vi "Get Configured Form Object.vi"(8 "error in (no error)":errorcluster, 10 "Table Name":string, 11 "Form from Table Configuration in":refnum<class "Form from Table Configuration.lvclass">) -> (0 "error out":errorcluster, 2 "Configured Form":refnum<class "Basic Form.lvclass">, 3 "Form from Table Configuration out":refnum<class "Form from Table Configuration.lvclass">)   [LabVIEW 2020, in "Panel Form Controller.lvlib" / "Form from Table Configuration.lvclass"]
uses:
  Form from Table Configuration.lvclass
  Database OOP/Table Libraries/Basic Form/Basic Form.lvclass
  Form from Table Configuration.lvclass/Form from Table Configuration.ctl
  Database OOP/Table Libraries/Table Configuration Interface/Table Configuration Interface.lvclass
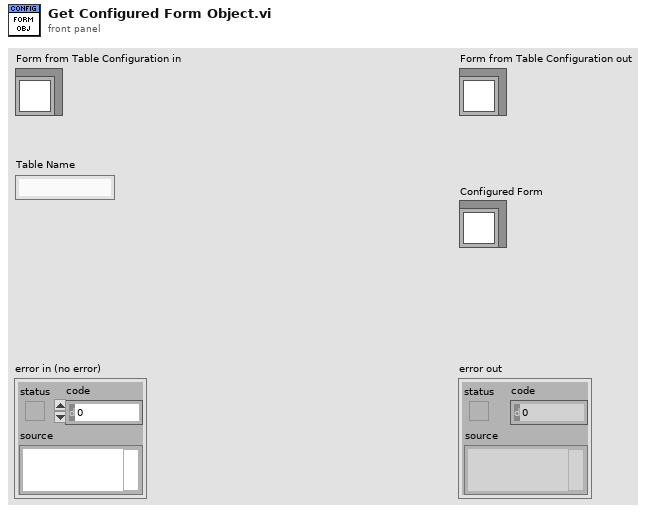
[diagram p1: front panel]
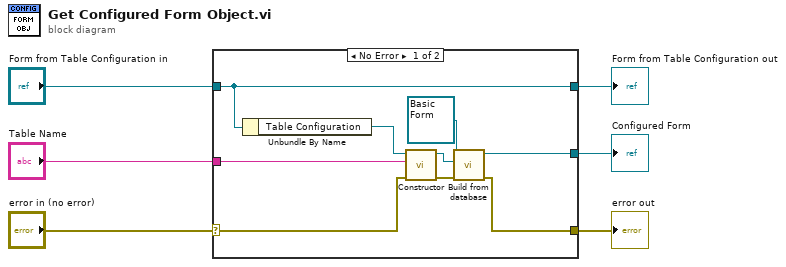
[diagram p0: block diagram]
diagram:
  n1 = case shown="No Error" "error in (no error)" {
    selector: "error in (no error)" -> [w8 w17]
    tunnel: [w7 w17] -> w5
    tunnel: "Form from Table Configuration in" -> [w15 w16]
    tunnel: [w15 w16] -> w3
    tunnel: "Table Name" -> [w13 _]
    tunnel: [w9 _] -> w1
    frame No Error {
      n2 = Unbundle By Name(w15) -> ("Table Configuration"=w14:refnum<class "Table Configuration Interface.lvclass">)
      n3 = call-dynamic "Constructor.vi"("error in (no error)"=w8, "Table Name (Use Member Data)"=w13, "Table Configuration Interface in"=w14) -> ("error out"=w12:errorcluster, "Table Configuration Interface out"=w11:refnum<class "Table Configuration Interface.lvclass">)  [unwired: 7 in]
      n4 = call-dynamic "Build from database.vi"("error in (no error)"=w12, "Table Configuration"=w11, "Table in"=refnum<class "Basic Form.lvclass"> refnum ("Configured Form")) -> ("error out"=w7:errorcluster, "Table out"=w9:refnum<class "Basic Form.lvclass">)  [unwired: 7 in]
    }
    frame Error {
    }
  }
  "error out" <- w5
  "Form from Table Configuration out" <- w3
  "Configured Form" <- w1
